vi "API String Config Global.vi"() -> ()   [LabVIEW 2017, in "API String Arguments Support.lvlib"]
uses:
  API String Arguments Support.lvlib
panel:
  out "API String Config Flag":u64=4603270806574966694 format="%08x"
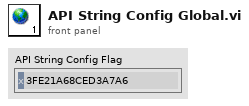
[diagram p1: front panel]
diagram:
